vi "Load Image.vi"(8 "error in (no error)":errorcluster, 9 "Image Index":i32=1, 10 "Image Data":T1, 11 "Image File":path) -> (0 "error out":errorcluster, 2 "Number Of Images":i32, 3 "Image":refnum<k24>)   [LabVIEW 2019]
doc: "This VI will load an image file into a PictureBox .Net control. The file it will load is the one provided by <B>Image File</B>. It will then display the image using the setting found in <B>Size Mode (Zoom)</B>. Zoom will make the picture fit the control while keeping the aspect ratio, while Stretch will fill the control in all directions.\n\nIf a file is not provided by <B>Image File</B>, the data found in <B>Image Data</B> will be used instead to display the image into the PictureBox.\n\nNote that the image does not stay in the PictureBox after the VI has stopped executing.\n\n-----\nBrian Hoover (hooovahh)"
uses:
  <vilib>/wsapi/NI_WebServices.lvlib
  System.Drawing
  <vilib>/picture/picture.llb/imagedata.ctl
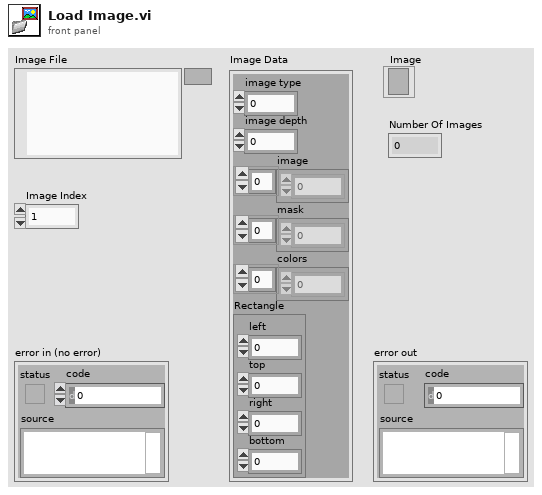
[diagram p1: front panel]
types:
  T1 = typedef "imagedata.ctl" = cluster{"image type":i32, "image depth":i32, "image":u8[], "mask":u8[], "colors":u32[], "Rectangle":cluster{"left":i16, "top":i16, "right":i16, "bottom":i16}}
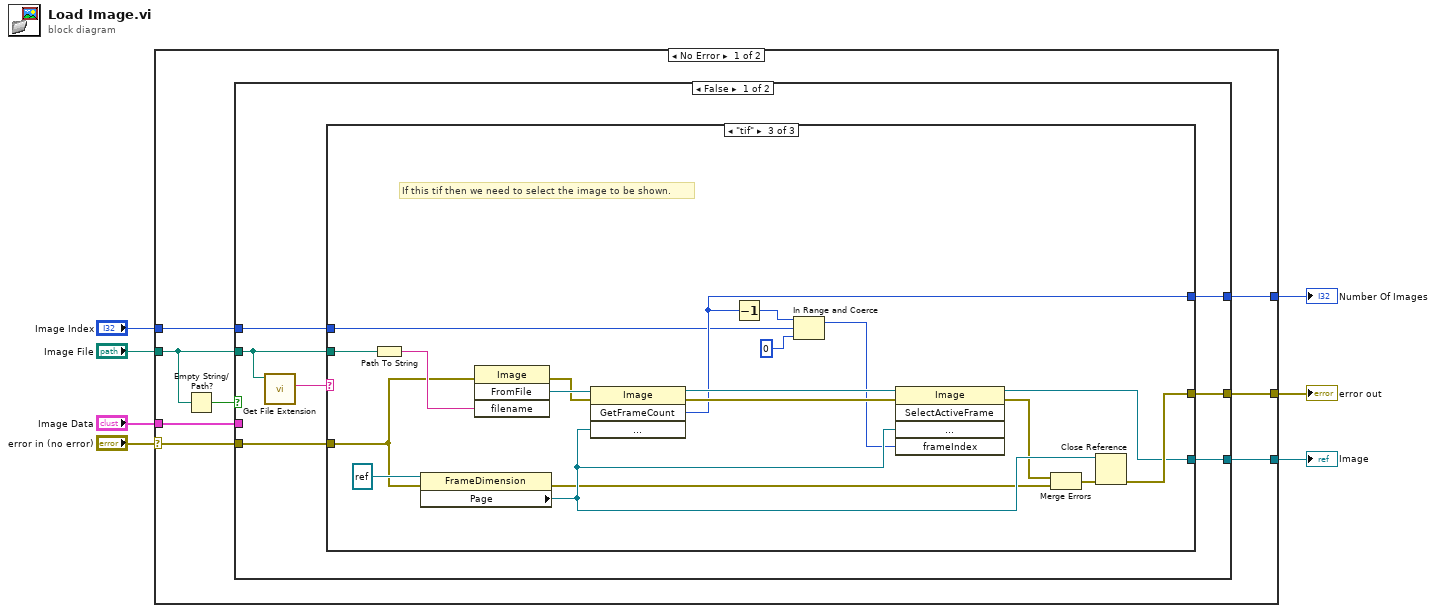
[diagram p0: block diagram]
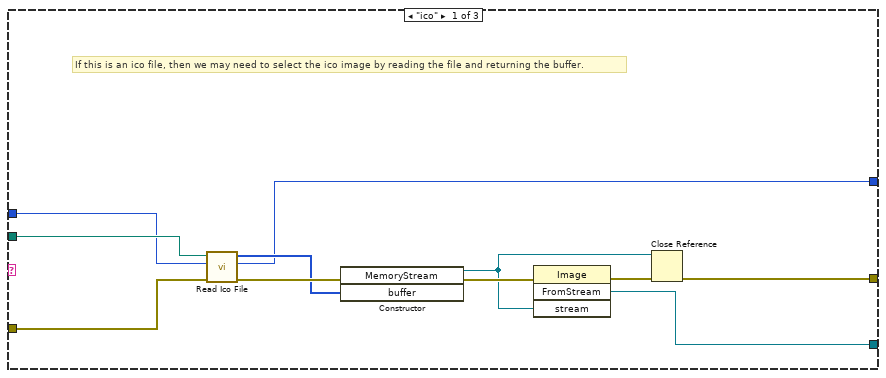
[diagram p2: hidden frame]
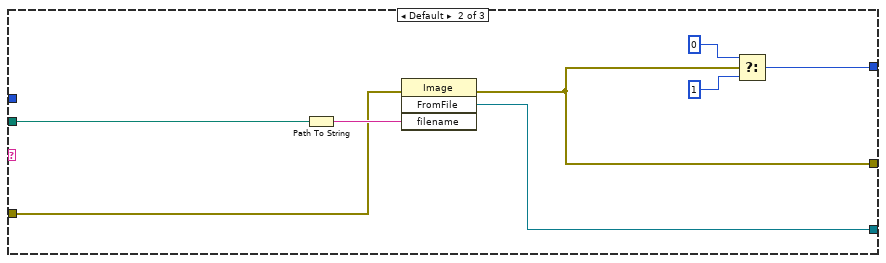
[diagram p3: hidden frame]
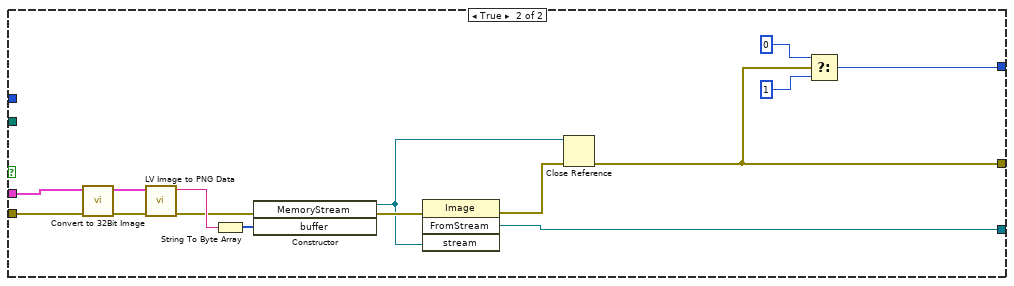
[diagram p4: hidden frame]
diagram:
  n1 = case shown="No Error" "error in (no error)" {
    selector: "error in (no error)" -> [w12 w76]
    tunnel: "Image Data" -> [w14 _]
    tunnel: "Image File" -> [w13 _]
    tunnel: [w11 _] -> w5
    tunnel: [w10 w76] -> w4
    tunnel: "Image Index" -> [w9 _]
    tunnel: [w8 _] -> w1
    frame No Error {
      n2 = Empty String/Path?(string/path=w13) -> (empty?=w15:bool)
      n3 = case shown="False" w15 {
        tunnel: w14 -> [_ w66]
        tunnel: w13 -> [w20 _]
        tunnel: w12 -> [w18 w65]
        tunnel: [w22 w69] -> w11
        tunnel: [w21 w64] -> w10
        tunnel: w9 -> [w17 _]
        tunnel: [w16 w61] -> w8
        frame False {
          n4 = call <vilib>:"Get File Extension.vi"("file"=w20) -> ("lowercase file extension"=w19:string)  [unwired: 6 in, 4 out]
          n5 = case shown="\"tif\"" w19 {
            tunnel: [w30 w41 w47] -> w22
            tunnel: [w31 w35 w48] -> w21
            tunnel: w20 -> [w29 w39 w55]
            tunnel: w18 -> [w28 w38 w53]
            tunnel: w17 -> [w25 _ w44]
            tunnel: [w23 w34 w45] -> w16
            frame "ico" {
              # "If this is an ico file, then we may need to select the ico image by reading the file and returning the buffer."
              n6 = call "Read Ico File.vi"("error in (no error)"=w28, "Image Index"=w25, "Ico File"=w29) -> ("error out"=w27:errorcluster, "Number Of Images"=w23:u16, "Byte Array"=w26:u8[])  [unwired: 6 in]
              n7 = constructor class="MemoryStream"(error in=w27, "buffer"=w26) -> (reference out=w24:refnum<k24>, error out=w33:errorcluster)  [unwired: 2 in, 2 out]
              n8 = invoke class="Image" method="FromStream"(error in=w33, "stream"=w24) -> (error out=w32:errorcluster, "FromStream"=w30:refnum<k24>)  [unwired: 2 in, 2 out]
              n9 = Close Reference(reference=w24, error in (no error)=w32) -> (error out=w31:errorcluster)
            }
            frame Default {
              n10 = Path To String(path=w39) -> (string=w40:string)
              n11 = invoke class="Image" method="FromFile"(error in=w38, "filename"=w40) -> (error out=w35:errorcluster, "FromFile"=w41:refnum<k24>)  [unwired: 2 in, 2 out]
              n12 = Select(t=0 ("GetFrameCount"), s=w35, f=1 ("GetFrameCount")) -> (s? t:f=w34:i32)
            }
            frame "tif" {
              # "If this tif then we need to select the image to be shown."
              n13 = Path To String(path=w55) -> (string=w54:string)
              n14 = property class="FrameDimension"(reference=refnum<k24> refnum ("dimension"), error in=w53) -> (error out=w49:errorcluster, "Page"=w59:refnum<k24>)  [unwired: 1 out]
              n15 = invoke class="Image" method="FromFile"(error in=w53, "filename"=w54) -> (error out=w52:errorcluster, "FromFile"=w56:refnum<k24>)  [unwired: 2 in, 2 out]
              n16 = invoke class="Image" method="GetFrameCount"(reference=w56, error in=w52, "dimension"=w59) -> (reference out=w60:refnum<k24>, error out=w58:errorcluster, "GetFrameCount"=w45:i32)  [unwired: 1 in, 1 out]
              n17 = Decrement(x=w45) -> (x-1=w42:i32)
              n18 = In Range and Coerce(upper limit=w42, x=w44, lower limit=0) -> (coerced(x)=w43:i32)  [unwired: 1 out]
              n19 = invoke class="Image" method="SelectActiveFrame"(reference=w60, error in=w58, "dimension"=w59, "frameIndex"=w43) -> (reference out=w47:refnum<k24>, error out=w50:errorcluster)  [unwired: 1 in, 3 out]
              n20 = Merge Errors(w50, w49) -> (w51:errorcluster)
              n21 = Close Reference(reference=w59, error in (no error)=w51) -> (error out=w48:errorcluster)
            }
          }
        }
        frame True {
          n22 = call "Convert to 32Bit Image.vi"("error in (no error)"=w65, "Image Data"=w66) -> ("error out"=w74:errorcluster, "32Bit Image Data Out"=w75:T1)  [unwired: 8 in]
          n23 = call <vilib>:"LV Image to PNG Data.vi"("error in (no error)"=w74, "image data"=w75) -> ("error out"=w71:errorcluster, "png data"=w72:string)  [unwired: 8 in]
          n24 = String To Byte Array(string=w72) -> (unsigned byte array=w73:u8[])
          n25 = constructor class="MemoryStream"(error in=w71, "buffer"=w73) -> (reference out=w68:refnum<k24>, error out=w70:errorcluster)  [unwired: 2 in, 2 out]
          n26 = invoke class="Image" method="FromStream"(error in=w70, "stream"=w68) -> (error out=w67:errorcluster, "FromStream"=w69:refnum<k24>)  [unwired: 2 in, 2 out]
          n27 = Close Reference(reference=w68, error in (no error)=w67) -> (error out=w64:errorcluster)
          n28 = Select(t=0 ("GetFrameCount"), s=w64, f=1 ("GetFrameCount")) -> (s? t:f=w61:i32)
        }
      }
    }
    frame Error {
    }
  }
  "error out" <- w4
  "Image" <- w5
  "Number Of Images" <- w1
